vi "UI_Elmts_Visible[Labels].vi"(8 "error in (no error)":errorcluster, 9 "Visible":bool, 10 "Elmts Labels":string[](array[string]), 11 "UI_Actor in":refnum<class "UI_Actor.lvclass">) -> (0 "error out":errorcluster, 1 "Founds":bool[](array[boolean]), 3 "UI_Actor out":refnum<class "UI_Actor.lvclass">)   [LabVIEW 2020, in "UI_Actor.lvlib" / "UI_Actor.lvclass"]
uses:
  UI_Actor.lvclass
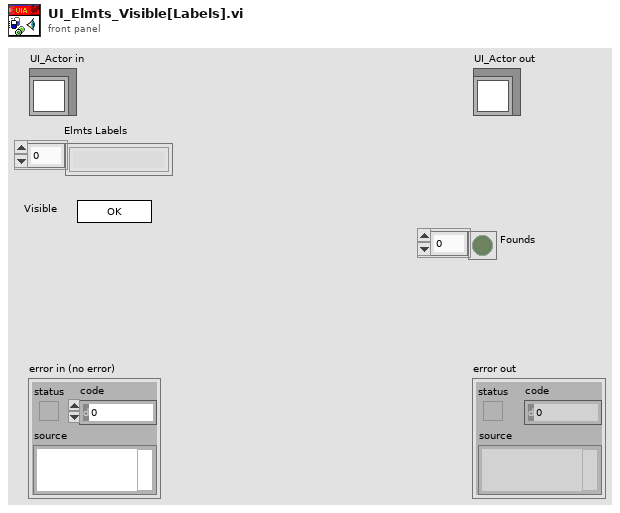
[diagram p1: front panel]
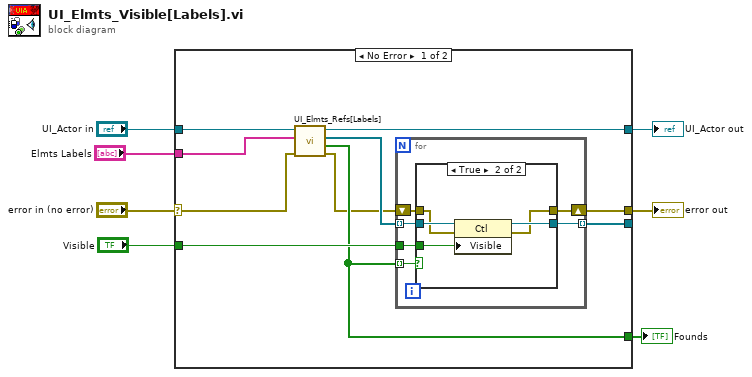
[diagram p0: block diagram]
diagram:
  n1 = case shown="No Error" "error in (no error)" {
    selector: "error in (no error)" -> [w12 w32]
    tunnel: [w17 w32] -> w6
    tunnel: [w11 w31] -> w4
    tunnel: "UI_Actor in" -> [w14 w31]
    tunnel: "Elmts Labels" -> [w13 _]
    tunnel: [w16 _] -> _
    tunnel: [w9 _] -> w2
    tunnel: "Visible" -> [w15 _]
    frame No Error {
      n2 = call "UI_Elmts_Refs[Labels].vi"("error in (no error)"=w12, "Elmts Labels"=w13, "UI_Actor in"=w14) -> ("error out"=w8:errorcluster, "Founds"=w9:bool[], "Refs"=w10:refnum<vi>[], "UI_Actor out"=w11:refnum<class "UI_Actor.lvclass">)  [unwired: 5 in]
      n3 = for {
        tunnel: [w22] -> w16 mode=indexing
        tunnel: w15 -> [w21]
        tunnel: w10 -> [w20] mode=indexing
        tunnel: w9 -> [w19] mode=indexing
        shift-right: [w23] -> w17
        shift-left: w8 -> [w18]
        n4 = case shown="True" w19 {
          tunnel: [w25 w30] -> w22
          tunnel: w20 -> [w25 w29]
          tunnel: w21 -> [_ w28]
          tunnel: w18 -> [w24 w27]
          tunnel: [w24 w26] -> w23
          frame False {
          }
          frame True {
            n5 = property class="Ctl"(reference=w29, error in=w27, "Visible"=w28) -> (reference out=w30:refnum<vi>, error out=w26:errorcluster)
          }
        }
      }
    }
    frame Error {
    }
  }
  "error out" <- w6
  "UI_Actor out" <- w4
  "Founds" <- w2
